vi "Init.vi"(0 "CSV Test Log in":refnum<class "CSV Test Log.lvclass">, 5 "Log Path":path, 7 "Test Name":string, 9 "Scan Name":string, 11 "error in (no error)":errorcluster) -> (4 "CSV Test Log out":refnum<class "CSV Test Log.lvclass">, 15 "error out":errorcluster)   [LabVIEW 2016, in "CSV Test Log.lvclass"]
uses:
  CSV Test Log.lvclass
  CSV Test Log.lvclass/CSV Test Log.ctl
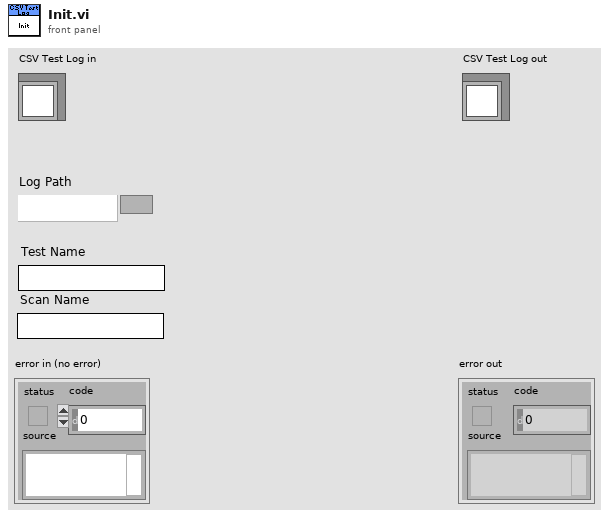
[diagram p1: front panel]
types:
  T1 = enum16{"open", "replace", "create", "open or create", "replace or create", "replace or create with confirmation"}
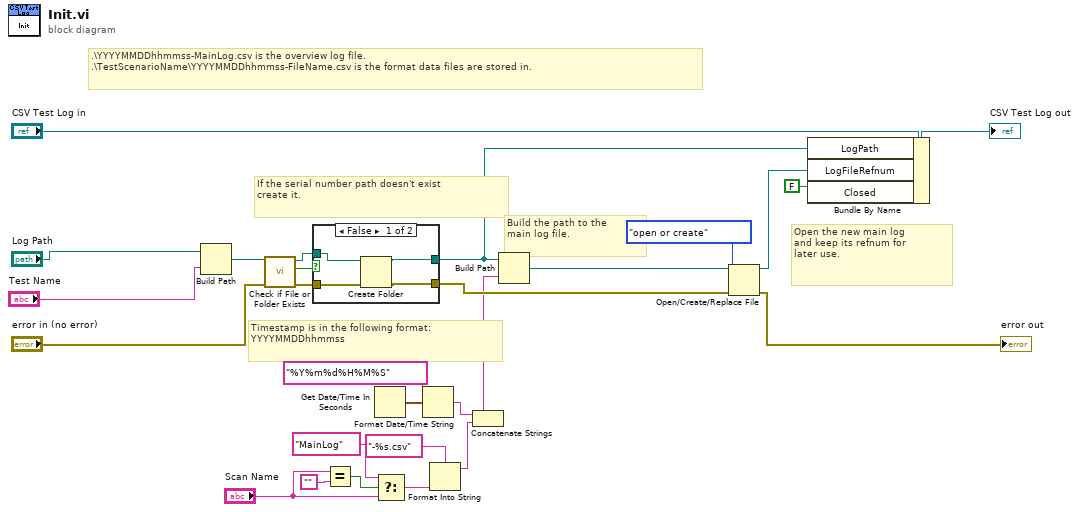
[diagram p0: block diagram]
diagram:
  # "Build the path to the\nmain log file."
  # "Open the new main log\nand keep its refnum for\nlater use."
  # "Timestamp is in the following format:\nYYYYMMDDhhmmss"
  # "If the serial number path doesn't exist\ncreate it."
  # ".\\YYYYMMDDhhmmss-MainLog.csv is the overview log file.\n.\\TestScenarioName\\YYYYMMDDhhmmss-FileName.csv is the format data files are stored in."
  n1 = Build Path(base path="Log Path", name or relative path="Test Name") -> (appended path=w22:path)
  n2 = call <vilib>:"Check if File or Folder Exists.vi"("error in (no error)"="error in (no error)", "path"=w22) -> ("error out"=w25:errorcluster, "file or folder exists?"=w23:bool, "dup path"=w24:path)  [unwired: 7 in]
  n3 = case shown="False" w23 {
    tunnel: w24 -> [w31 w33]
    tunnel: w25 -> [w30 w32]
    tunnel: [w29 w32] -> w26
    tunnel: [w28 w33] -> w27
    frame False {
      n4 = Create Folder(path (use dialog)=w31, error in=w30) -> (created path=w28:path, error out=w29:errorcluster)  [unwired: 1 in, 1 out]
    }
    frame True {
    }
  }
  n5 = Equal?(x="Scan Name", y="") -> (x = y?=w5:bool)
  n6 = Get Date/Time In Seconds() -> (seconds since 1Jan1904=w17:timestamp)
  n7 = Select(t="MainLog" ("string"), s=w5, f="Scan Name") -> (s? t:f=w2:string)
  n8 = Format Date/Time String(time format string (%c)="%Y%m%d%H%M%S", seconds (now)=w17) -> (date/time string=w19:string)  [unwired: 1 in]
  n9 = Format Into String(format string="-%s.csv", w2) -> (resulting string=w1:string)  [unwired: 2 in, 1 out]
  n10 = Concatenate Strings(w19, w1) -> (w15:string)
  n11 = Build Path(base path=w27, name or relative path=w15) -> (appended path=w20:path)
  n12 = Open/Create/Replace File(file path (use dialog)=w20, error in=w26, operation (0:open)=T1."open or create") -> (refnum out=w21:refnum<file>, error out=→"error out":errorcluster)  [unwired: 3 in, 1 out]
  n13 = Bundle By Name(cluster="CSV Test Log in", "LogPath"=w27, "LogFileRefnum"=w21, "Closed"=FALSE) -> (→"CSV Test Log out":refnum<class "CSV Test Log.lvclass">)
